vi "Flywheel_Execute.vi"() -> ()   [LabVIEW 2019]
uses:
  Utility_VIs/Basic_Motor_Modes.ctl
  Flywheel_Globals.vi
  Sensing/Sensor_Values.vi
panel:
  in  "array 2":dbl[][](array[numeric])
  in  "array":dbl[][](array[numeric])
  out "added Area":dbl=-0.27951836585998535
  in  "Camera Area D":dbl=17.0
  in  "Default_Flywheel_Speed":dbl=4750.0
  in  "Flywheel_MaxSpeed":dbl=16000.0
  out "Camera_Area":dbl=1.2052602767944336
  out "Error":cluster{dbl, dbl}(graph)
  out "Spun-Up":bool
  out "Error":dbl
  in  "Acceptable_error":dbl=200.0
  # "Click here to set min"
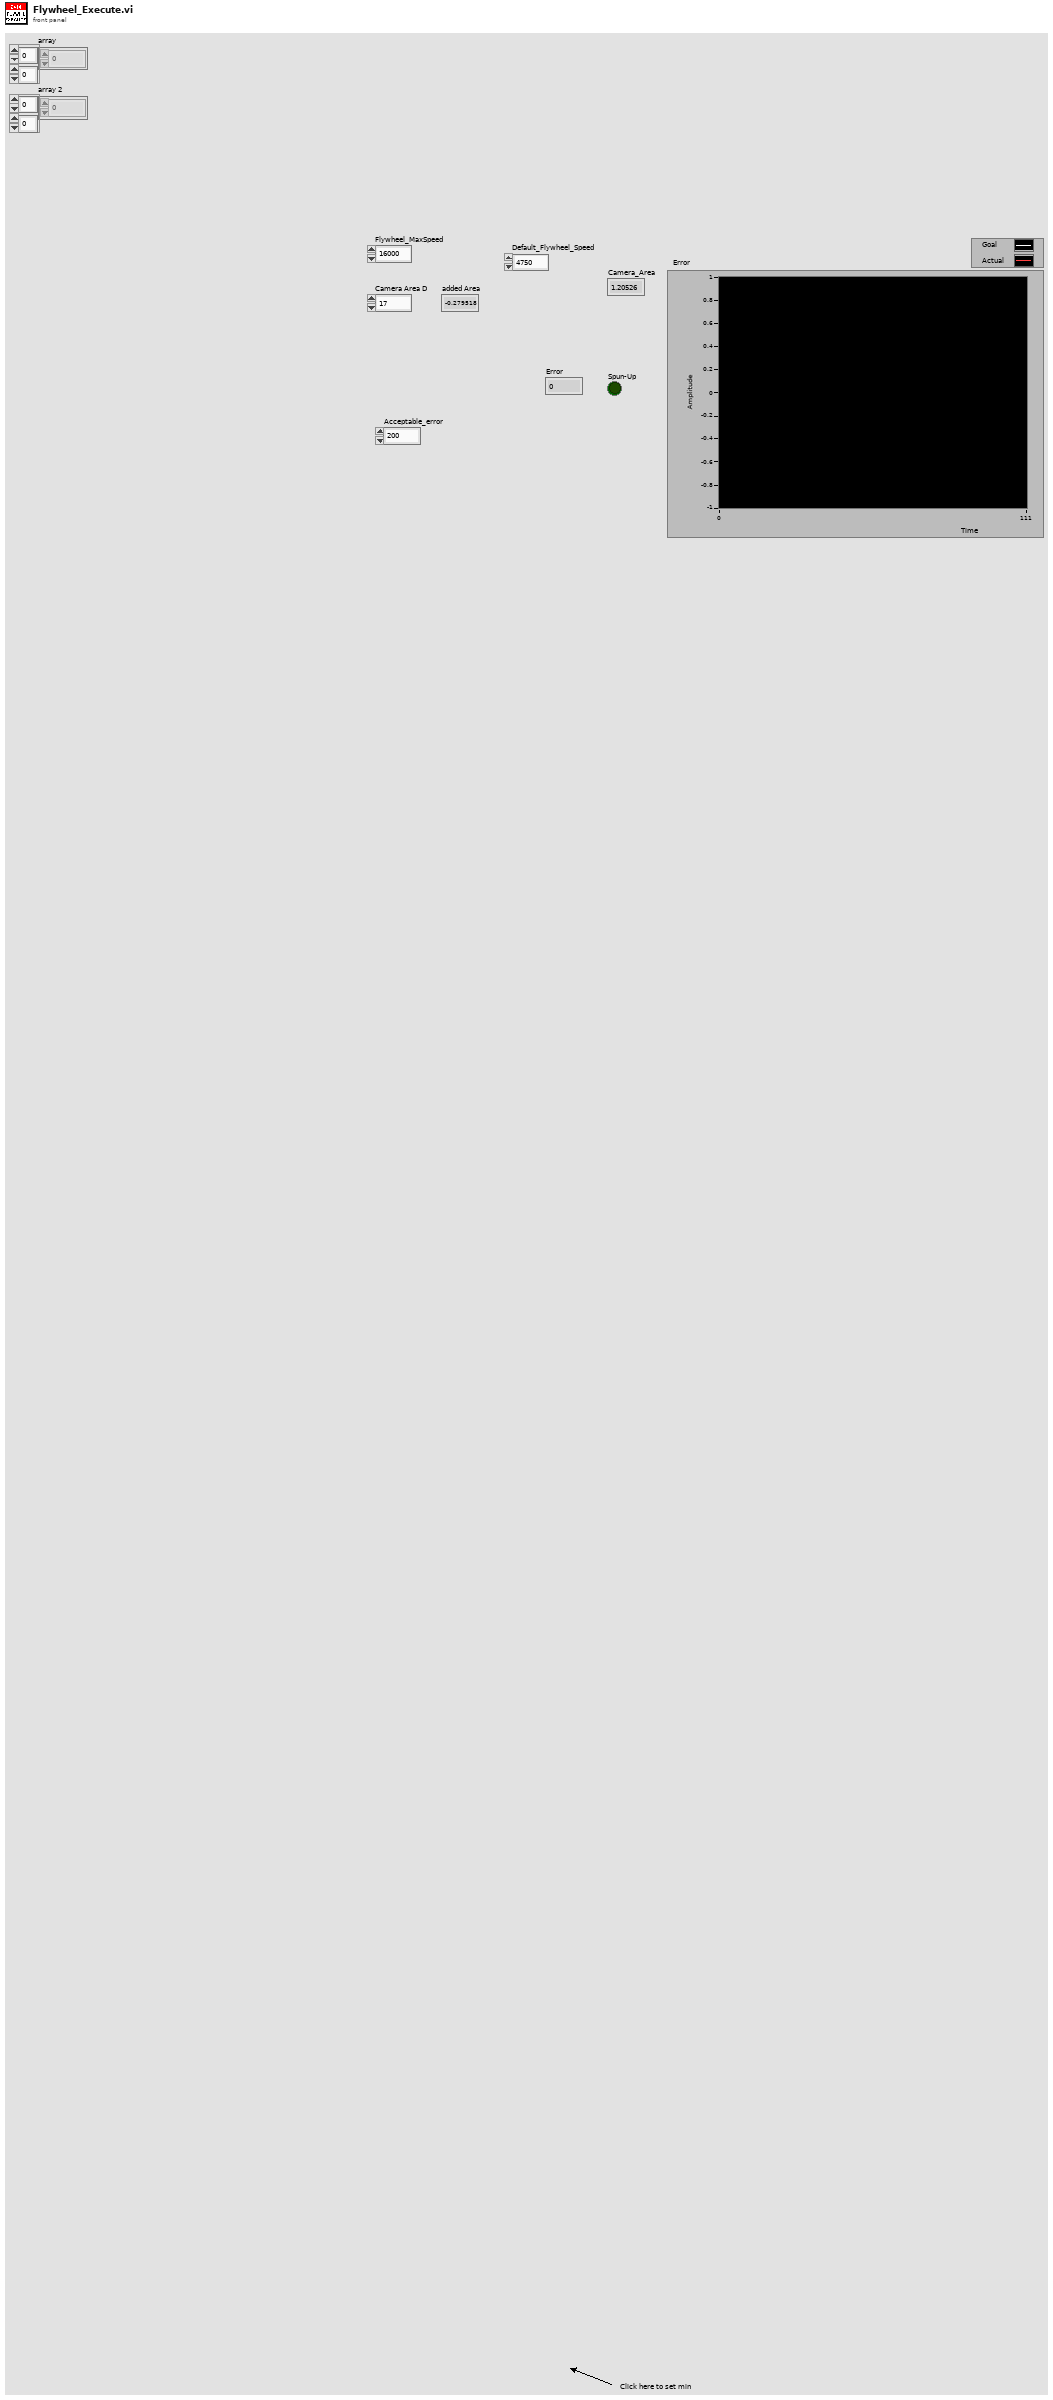
[diagram p1: front panel]
types:
  T1 = typedef "Basic_Motor_Modes.ctl" = enum16{"Percent_Voltage", "Speed_Control", "Position_Control", "Current"}
  T2 = typedef "Flywheel_Cluster.ctl" = cluster{"Flywheel_Throttle":dbl, "Control_States":T3, "Auto_Speed":bool, "Flywheel_On":bool, "Parameter_1":dbl, "Parameter_2":dbl, "Auto_Notifier":refnum<notifier>, "Step":dbl}
  T3 = typedef "Flywheel_States.ctl" = enum16{"No-Op", "Percent_Voltage", "Speed_Control_Manual", "Speed_Control_Auto", "Command_SpinUp", "Command_SpinUpAuto"}
  T4 = cluster{"Flywheel_Output":dbl, "Flywheel_Velocity(RPM)":dbl}
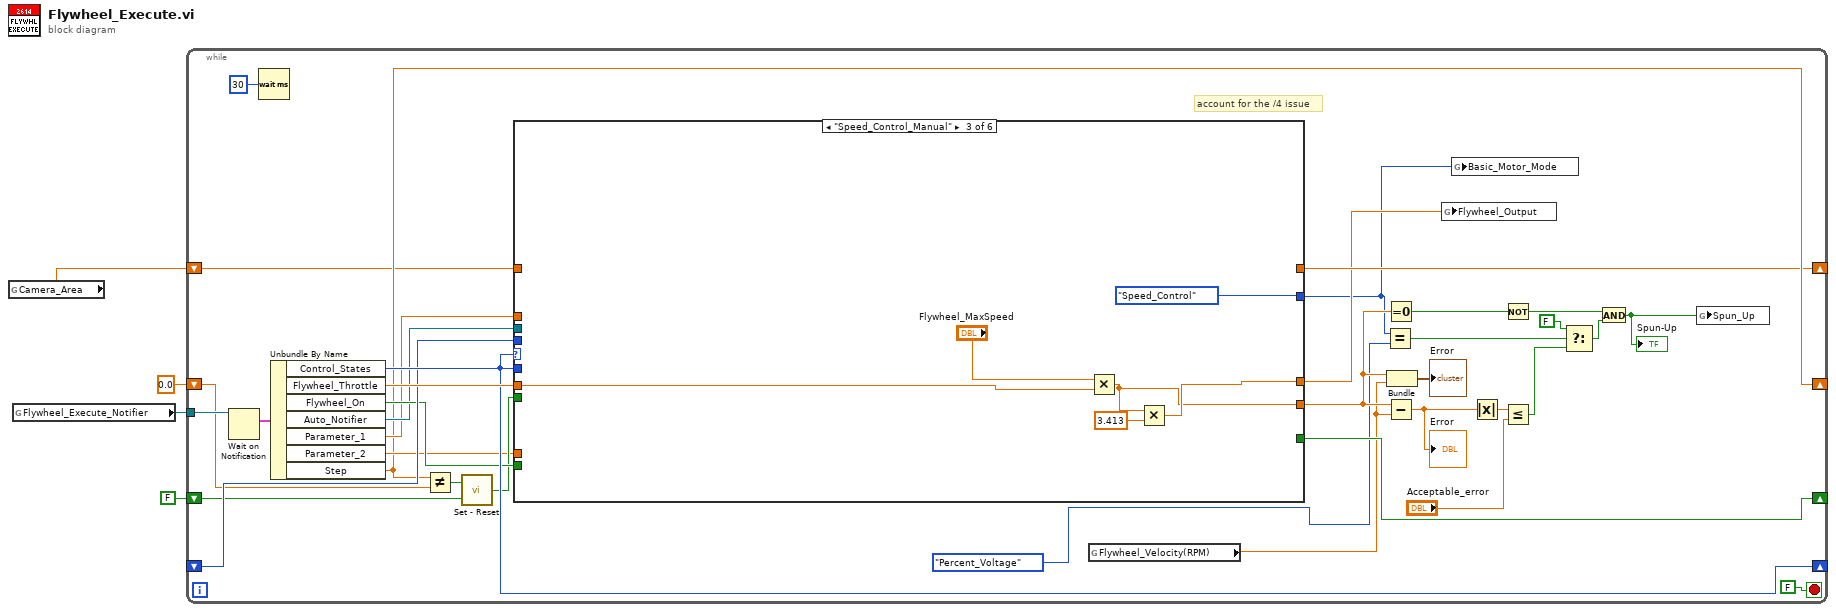
[diagram p0: block diagram]
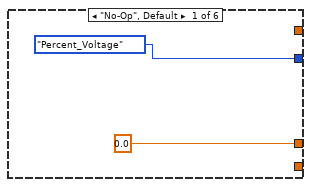
[diagram p2: hidden frame]
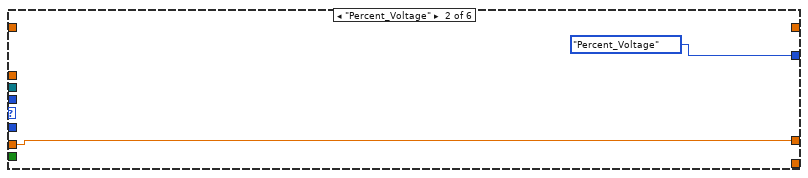
[diagram p3: hidden frame]
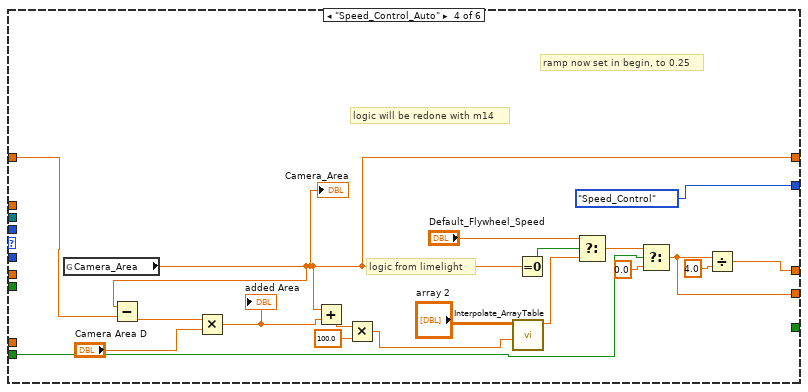
[diagram p4: hidden frame]
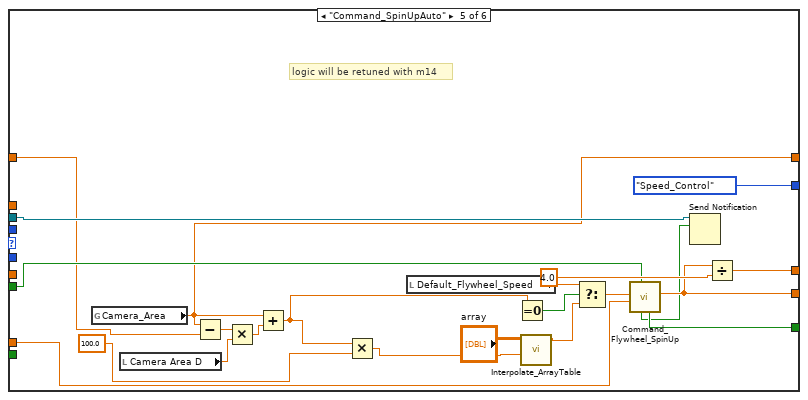
[diagram p5: hidden frame]
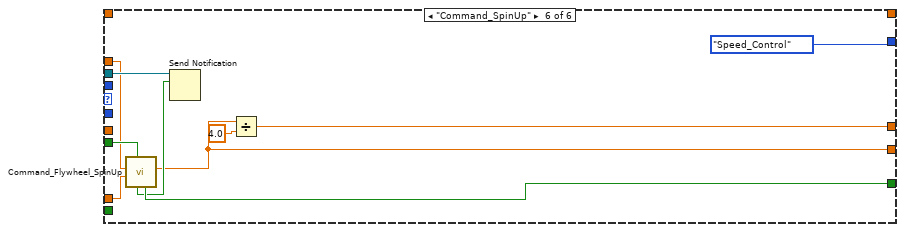
[diagram p6: hidden frame]
diagram:
  n1 = global read "Sensor_Values.vi" "Camera_Area"() -> (w1:dbl)
  n2 = global read "Flywheel_Globals.vi" "Flywheel_Execute_Notifier"() -> (w4:refnum<notifier>)
  n3 = while {
    tunnel: w4 -> [w38]
    shift-right: [w34] -> _
    shift-left: _ -> [w33]
    shift-right: [w12] -> _
    shift-left: 0.0 ("Step") -> [w11]
    shift-right: [w17] -> _
    shift-left: FALSE ("Reint") -> [w18]
    shift-right: [w9] -> _
    shift-left: w1 -> [w10]
    stop <- FALSE stop-if-true
    # "account for the /4 issue"
    n4 = Wait on Notification(notifier=w38) -> (notification=w37:T2)  [unwired: 3 in, 3 out]
    n5 = Wait (ms)(milliseconds to wait=u32 30) -> ()  [unwired: 1 out]
    n6 = Unbundle By Name(w37) -> ("Control_States"=w34:T3, "Flywheel_Throttle"=w36:dbl, "Flywheel_On"=w22:bool, "Auto_Notifier"=w16:refnum<notifier>, "Parameter_1"=w15:dbl, "Parameter_2"=w14:dbl, "Step"=w12:dbl)
    n7 = Not Equal?(x=w12, y=w11) -> (x != y?=w13:bool)
    n8 = call "Set - Reset.vi"("Reset"=w18, "Set"=w13) -> ("Output"=w19:bool)
    n9 = case shown="\"Speed_Control_Manual\"" w34 {
      tunnel: [0.0 ("Flywheel_Throttle") w43 w47 w68 w89 w94] -> w8
      tunnel: w36 -> [_ w43 w49 _ _ _]
      tunnel: w34 -> [_ _ _ _ _ _]
      tunnel: w33 -> [_ _ _ _ _ _]
      tunnel: [_ _ w44 w67 w84 w92] -> w24
      tunnel: w22 -> [_ _ _ w66 _ _]
      tunnel: w19 -> [_ _ _ _ w82 w100]
      tunnel: [_ _ _ _ w81 w99] -> w17
      tunnel: w16 -> [_ _ _ _ w80 w98]
      tunnel: w15 -> [_ _ _ _ _ w96]
      tunnel: w14 -> [_ _ _ _ w83 w95]
      tunnel: w10 -> [_ _ _ w58 w71 _]
      tunnel: [_ _ _ w53 w75 _] -> w9
      tunnel: [Basic_Motor_Modes."Percent_Voltage" ("Motor_Mode") Basic_Motor_Modes."Percent_Voltage" ("Motor_Mode") Basic_Motor_Modes."Speed_Control" ("Motor_Mode") Basic_Motor_Modes."Speed_Control" ("Motor_Mode") Basic_Motor_Modes."Speed_Control" ("Motor_Mode") Basic_Motor_Modes."Speed_Control" ("Motor_Mode")] -> w6
      frame "No-Op", Default {
      }
      frame "Percent_Voltage" {
      }
      frame "Speed_Control_Manual" {
        n10 = Multiply(x="Flywheel_MaxSpeed", y=w49) -> (x*y=w44:dbl)
        n11 = Multiply(x=w44, y=3.413) -> (x*y=w47:dbl)
      }
      frame "Speed_Control_Auto" {
        # "logic will be redone with m14"
        # "ramp now set in begin, to 0.25"
        # "logic from limelight"
        n12 = global read "Sensor_Values.vi" "Camera_Area"() -> (w53:dbl)
        "Camera_Area" <- w53
        n13 = Subtract(x=w53, y=w58) -> (x-y=w57:dbl)
        n14 = Multiply(x=w57, y="Camera Area D") -> (x*y=w52:dbl)
        "added Area" <- w52
        n15 = Add(x=w53, y=w52) -> (x+y=w54:dbl)
        n16 = Multiply(x=w54, y=100.0) -> (x*y=w59:dbl)
        n17 = call "Interpolate_ArrayTable.vi"("Desired_Distance"=w59, "array"="array 2") -> ("RPM"=w60:dbl)  [unwired: 9 in]
        n18 = Equal To 0?(x=w53) -> (x = 0?=w63:bool)
        n19 = Select(t="Default_Flywheel_Speed", s=w63, f=w60) -> (s? t:f=w61:dbl)
        n20 = Select(t=w61, s=w66, f=0.0) -> (s? t:f=w67:dbl)
        n21 = Divide(x=w67, y=4.0) -> (x/y=w68:dbl)
      }
      frame "Command_SpinUpAuto" {
        # "logic will be retuned with m14"
        n22 = global read "Sensor_Values.vi" "Camera_Area"() -> (w75:dbl)
        n23 = local read "Camera Area D"() -> (w72:dbl)
        n24 = Subtract(x=w75, y=w71) -> (x-y=w74:dbl)
        n25 = Multiply(x=w74, y=w72) -> (x*y=w73:dbl)
        n26 = Add(x=w75, y=w73) -> (x+y=w76:dbl)
        n27 = Multiply(x=w76, y=100.0) -> (x*y=w77:dbl)
        n28 = local read "Default_Flywheel_Speed"() -> (w86:dbl)
        n29 = Equal To 0?(x=w76) -> (x = 0?=w87:bool)
        n30 = call "Interpolate_ArrayTable.vi"("Desired_Distance"=w77, "array"="array") -> ("RPM"=w78:dbl)  [unwired: 9 in]
        n31 = Select(t=w86, s=w87, f=w78) -> (s? t:f=w85:dbl)
        n32 = call "Command_Flywheel_SpinUp.vi"("Startup"=w82, "Timeout"=w83, "Speed"=w85) -> ("Flywheel_Output"=w84:dbl, "Reint"=w81:bool, "Completed"=w79:bool)  [unwired: 6 in]
        n33 = Send Notification(notification=w79, notifier=w80) -> ()  [unwired: 1 in, 2 out]
        n34 = Divide(x=w84, y=4.0) -> (x/y=w89:dbl)
      }
      frame "Command_SpinUp" {
        n35 = call "Command_Flywheel_SpinUp.vi"("Startup"=w100, "Timeout"=w95, "Speed"=w96) -> ("Flywheel_Output"=w92:dbl, "Reint"=w99:bool, "Completed"=w97:bool)  [unwired: 6 in]
        n36 = Send Notification(notification=w97, notifier=w98) -> ()  [unwired: 1 in, 2 out]
        n37 = Divide(x=w92, y=4.0) -> (x/y=w94:dbl)
      }
    }
    n38 = global read "Sensor_Values.vi" "Flywheel_Velocity(RPM)"() -> (w5:dbl)
    n39 = Equal?(x=w6, y=Basic_Motor_Modes."Percent_Voltage" ("Motor_Mode")) -> (x = y?=w30:bool)
    n40 = Equal To 0?(x=w24) -> (x = 0?=w27:bool)
    n41 = Subtract(x=w24, y=w5) -> (x-y=w25:dbl)
    "Error" <- w25
    n42 = Bundle("Flywheel_Output"=w24, "Flywheel_Velocity(RPM)"=w5) -> (→"Error":T4)  [unwired: 1 in]
    n43 = global write "Flywheel_Globals.vi" "Flywheel_Output"(w8) -> ()
    n44 = global write "Flywheel_Globals.vi" "Basic_Motor_Mode"(w6) -> ()
    n45 = Absolute Value(x=w25) -> (abs(x)=w32:dbl)
    n46 = Not(x=w27) -> (.not. x?=w26:bool)
    n47 = Less Or Equal?(x=w32, y="Acceptable_error") -> (x <= y?=w28:bool)
    n48 = Select(t=FALSE, s=w30, f=w28) -> (s? t:f=w21:bool)
    n49 = And(x=w26, y=w21) -> (x .and. y?=w20:bool)
    "Spun-Up" <- w20
    n50 = global write "Flywheel_Globals.vi" "Spun_Up"(w20) -> ()
  }
